vi "gentec-SOLO-PE.Queries with String Answers.vi"(8 "error in (no error)":errorcluster, 10 "Queries with String Answers":T1="Version", 11 "VISA Refnum in":refnum<visa-resource-name>) -> (0 "error out":errorcluster, 1 "Answer":string, 2 "Error":string, 3 "VISA Refnum out":refnum<visa-resource-name>, 4 "Timeout":bool)   [LabVIEW 2014, in "gentec-SOLO-PE - Driver.lvlib"]
doc: "Queries the Head Name and the Firmware Version."
uses:
  gentec-SOLO-PE - Driver.lvlib
  Type Defs/gentec-SOLO-PE.Queries with String Answers.ctl
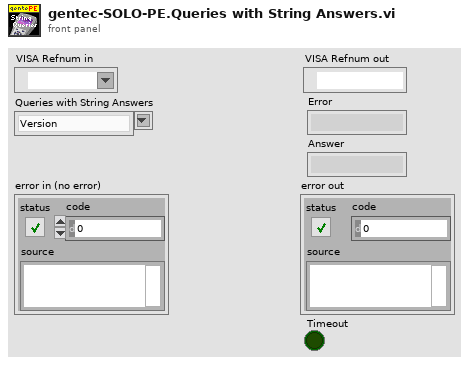
[diagram p1: front panel]
types:
  T1 = typedef "gentec-SOLO-PE - Driver.lvlib/gentec-SOLO-PE.Queries with String Answers.ctl" = string
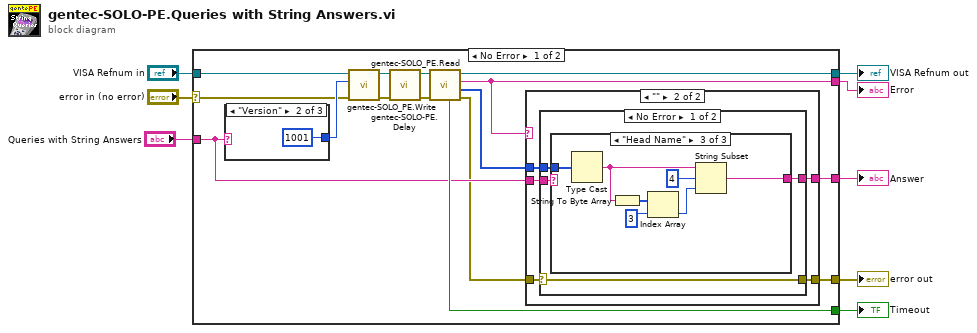
[diagram p0: block diagram]
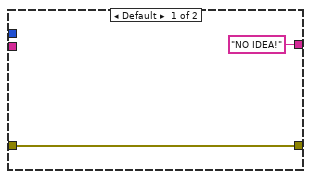
[diagram p2: hidden frame]
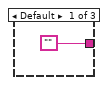
[diagram p3: hidden frame]
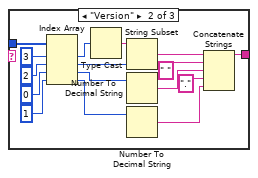
[diagram p4: hidden frame]
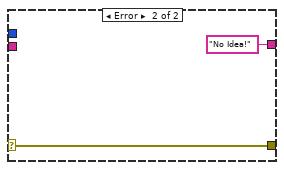
[diagram p5: hidden frame]
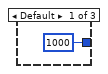
[diagram p6: hidden frame]
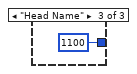
[diagram p7: hidden frame]
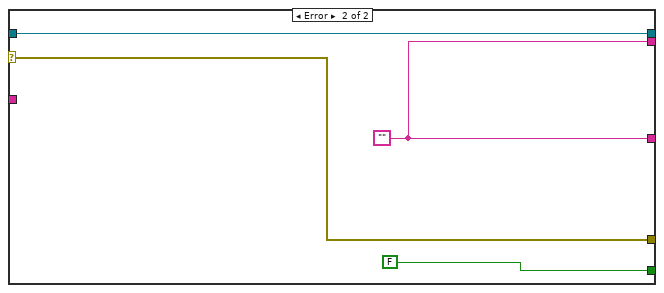
[diagram p8: hidden frame]
diagram:
  n1 = case shown="No Error" "error in (no error)" {
    selector: "error in (no error)" -> [w13 w65]
    tunnel: [w10 w65] -> w8
    tunnel: [w23 w67] -> w7
    tunnel: [w9 w66] -> w6
    tunnel: [w22 FALSE ("Timeout")] -> w5
    tunnel: "VISA Refnum in" -> [w17 w67]
    tunnel: [w15 w66] -> w3
    tunnel: "Queries with String Answers" -> [w14 _]
    frame No Error {
      n2 = case shown="\"Version\"" w14 {
        tunnel: [u16 1000 ("Command Handle") u16 1001 ("Command Handle") u16 1100 ("Command Handle")] -> w16
        frame Default {
        }
        frame "Version" {
        }
        frame "Head Name" {
        }
      }
      n3 = call "gentec-SOLO_PE.Write.vi"("error in (no error)"=w13, "Command Handle"=w16, "VISA Refnum in"=w17) -> ("error out"=w20:errorcluster, "VISA Refnum out"=w18:refnum<visa-resource-name>)  [unwired: 7 in]
      n4 = call "gentec-SOLO-PE.Delay.vi"("error in (no error)"=w20, "VISA resource In"=w18) -> ("error out"=w21:errorcluster, "VISA resource Out"=w19:refnum<visa-resource-name>)  [unwired: 4 in]
      n5 = call "gentec-SOLO_PE.Read.vi"("error in (no error)"=w21, "VISA Refnum in"=w19) -> ("error out"=w11:errorcluster, "Return Parameters"=w12:u32[], "Error"=w9:string, "VISA Refnum out"=w23:refnum<visa-resource-name>, "Timeout"=w22:bool)  [unwired: 5 in]
      n6 = case shown="\"\"" w9 {
        tunnel: ["NO IDEA!" w30] -> w15
        tunnel: w14 -> [_ w29]
        tunnel: w12 -> [_ w28]
        tunnel: w11 -> [w24 w27]
        tunnel: [w24 w26] -> w10
        frame Default {
        }
        frame "" {
          n7 = case shown="No Error" w27 {
            selector: w27 -> [w31 w59]
            tunnel: [w34 "No Idea!"] -> w30
            tunnel: w29 -> [w33 _]
            tunnel: w28 -> [w32 _]
            tunnel: [w31 w59] -> w26
            frame No Error {
              n8 = case shown="\"Head Name\"" w33 {
                tunnel: ["" w50 w54] -> w34
                tunnel: w32 -> [_ w36 w53]
                frame Default {
                }
                frame "Version" {
                  n9 = Index Array(array=w36, index #1=3 ("index"), index #2=2 ("index"), index #3=0 ("index"), index #4=1 ("index")) -> (element #1=w45:u32, element #2=w43:u32, element #3=w38:u32, element #4=w37:u32)
                  n10 = Type Cast(x=w45) -> (*(type *) &x=w44:string)  [unwired: 1 in]
                  n11 = String Subset(string=w44, length (rest)=w43) -> (substring=w51:string)  [unwired: 1 in]
                  n12 = Number To Decimal String(number=w38) -> (decimal integer string=w48:string)  [unwired: 1 in]
                  n13 = Number To Decimal String(number=w37) -> (decimal integer string=w46:string)  [unwired: 1 in]
                  n14 = Concatenate Strings(w51, " " ("string"), w48, "." ("string"), w46) -> (w50:string)
                }
                frame "Head Name" {
                  n15 = Type Cast(x=w53) -> (*(type *) &x=w52:string)  [unwired: 1 in]
                  n16 = String To Byte Array(string=w52) -> (unsigned byte array=w58:u8[])
                  n17 = Index Array(array=w58, index=3) -> (element=w57:u8)
                  n18 = String Subset(string=w52, offset (0)=4, length (rest)=w57) -> (substring=w54:string)
                }
              }
            }
            frame Error {
            }
          }
        }
      }
    }
    frame Error {
      w66 = ""
    }
  }
  "error out" <- w8
  "VISA Refnum out" <- w7
  "Error" <- w6
  "Timeout" <- w5
  "Answer" <- w3
